vi "sprawdzRuchPoziomy.vi"(8 "Wybór komory":T1, 9 "LINX Error IN":errorcluster, 10 "Czy nastapil krok?":bool, 11 "Stan poziomy":T2) -> (1 "LINX Error OUT":errorcluster, 2 "KONIEC":bool, 3 "Stan poziomy wybrany":T2=enum."WYŁ.")   [LabVIEW 2014]
uses:
  RuchPoziomy.ctl
  parametryKomorVIs/WyborKomory.ctl
  timerRuchuPoziomegoVIs/Czynnosc.ctl
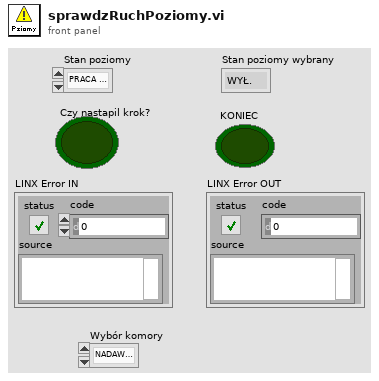
[diagram p1: front panel]
types:
  T1 = typedef "WyborKomory.ctl" = enum16{"NADAWCZA", "ODBIORCZA"}
  T2 = typedef "RuchPoziomy.ctl" = enum16{"PRACA RĘCZNA", "LEWO", "PRAWO", "WYŁ."}
  T3 = typedef "Czynnosc.ctl" = enum16{"reset all", "działaj"}
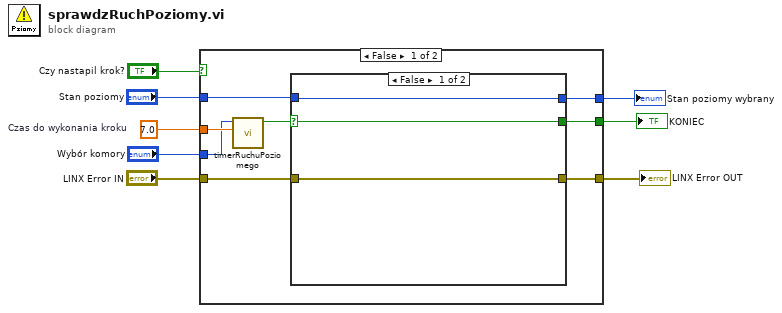
[diagram p0: block diagram]
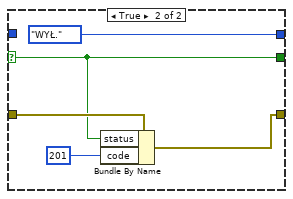
[diagram p2: hidden frame]
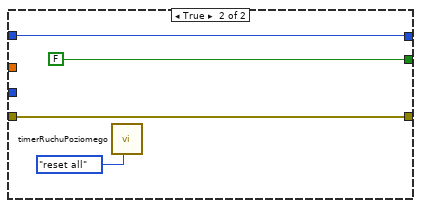
[diagram p3: hidden frame]
diagram:
  w6 = 7.0  # Czas do wykonania kroku
  n1 = case shown="False" "Czy nastapil krok?" {
    tunnel: "Stan poziomy" -> [w14 w27]
    tunnel: w6 -> [w16 _]
    tunnel: [w13 w27] -> w5
    tunnel: [w12 FALSE] -> w4
    tunnel: "LINX Error IN" -> [w11 w25]
    tunnel: [w10 w25] -> w2
    tunnel: "Wybór komory" -> [w9 _]
    frame False {
      n2 = call "timerRuchuPoziomego.vi"("Czas"=w16, "Wybór komory"=w9) -> ("Czy czas upłynął?"=w15:bool)  [unwired: 9 in]
      n3 = case shown="False" w15 {
        selector: w15 -> [w18 w21]
        tunnel: w14 -> [w19 _]
        tunnel: [w19 RuchPoziomy."WYŁ." ("Stan poziomy")] -> w13
        tunnel: [w18 w21] -> w12
        tunnel: w11 -> [w17 w23]
        tunnel: [w17 w22] -> w10
        frame False {
        }
        frame True {
          n4 = Bundle By Name(cluster=w23, "status"=w21, "code"=201 ("LINX Error Code")) -> (w22:errorcluster)
        }
      }
    }
    frame True {
      n5 = call "timerRuchuPoziomego.vi"("Czynność"=Czynnosc."reset all") -> ()  [unwired: 10 in, 1 out]
    }
  }
  "Stan poziomy wybrany" <- w5
  "KONIEC" <- w4
  "LINX Error OUT" <- w2
